vi "DuelistDirectIndirect.vi"(8 "error in (no error)":errorcluster, 10 "Game in":refnum<class "Game.lvclass">, 11 "NormalDefensiveWithDuelistPlay in":refnum<class "NormalDefensiveWithDuelistPlay.lvclass">) -> (0 "error out":errorcluster, 2 "duelist ?":bool, 3 "NormalDefensiveWithDuelistPlay out":refnum<class "NormalDefensiveWithDuelistPlay.lvclass">)   [LabVIEW 2018, in "NormalDefensiveWithDuelistPlay.lvclass"]
uses:
  NormalDefensiveWithDuelistPlay.lvclass
  Game_class/Game.lvclass
  Referee_class/command_interpreted.ctl
  Game_class/Game.lvclass/Game.ctl
  Referee_class/Referee.lvclass/Referee.ctl
  Events_class/Events.lvclass/Events.ctl
  Game_class/Read Referee.vi
  Game_class/Read EventsRef.vi
  Events_class/Read touch.vi
  Referee_class/Read command_interpreted.vi
  Referee_class/Referee.lvclass
  Events_class/Events.lvclass
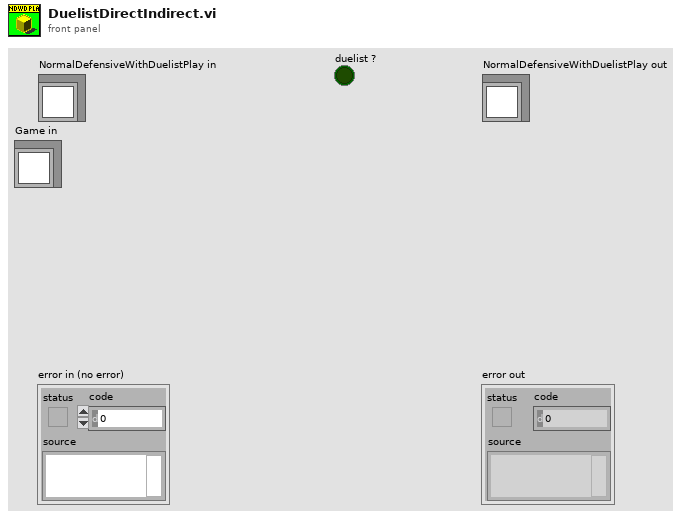
[diagram p1: front panel]
types:
  T1 = typedef "command_interpreted.ctl" = enum16{"Goal Ally", "Goal Enemy", "Ball Placement Enemy", "Ball Placement Ally", "Normal Half Time", "Extra Time  Break", "Extra Half Time", "None", "Post Game", "PKA Normal Start", "Prepare Kickoff Ally", "PKE Normal Start", "Prepare Kickoff Enemy", "Force Start", "Halt", "Timeout", "Prepare Penalty Ally", "Prepare Penalty Enemy", "PPA NormalStart", "PPE Normal Start", "Indirect Free Ally", "Direct Free Enemy", "Direct Free Ally", "Indirect Free Enemy", "Stop"}
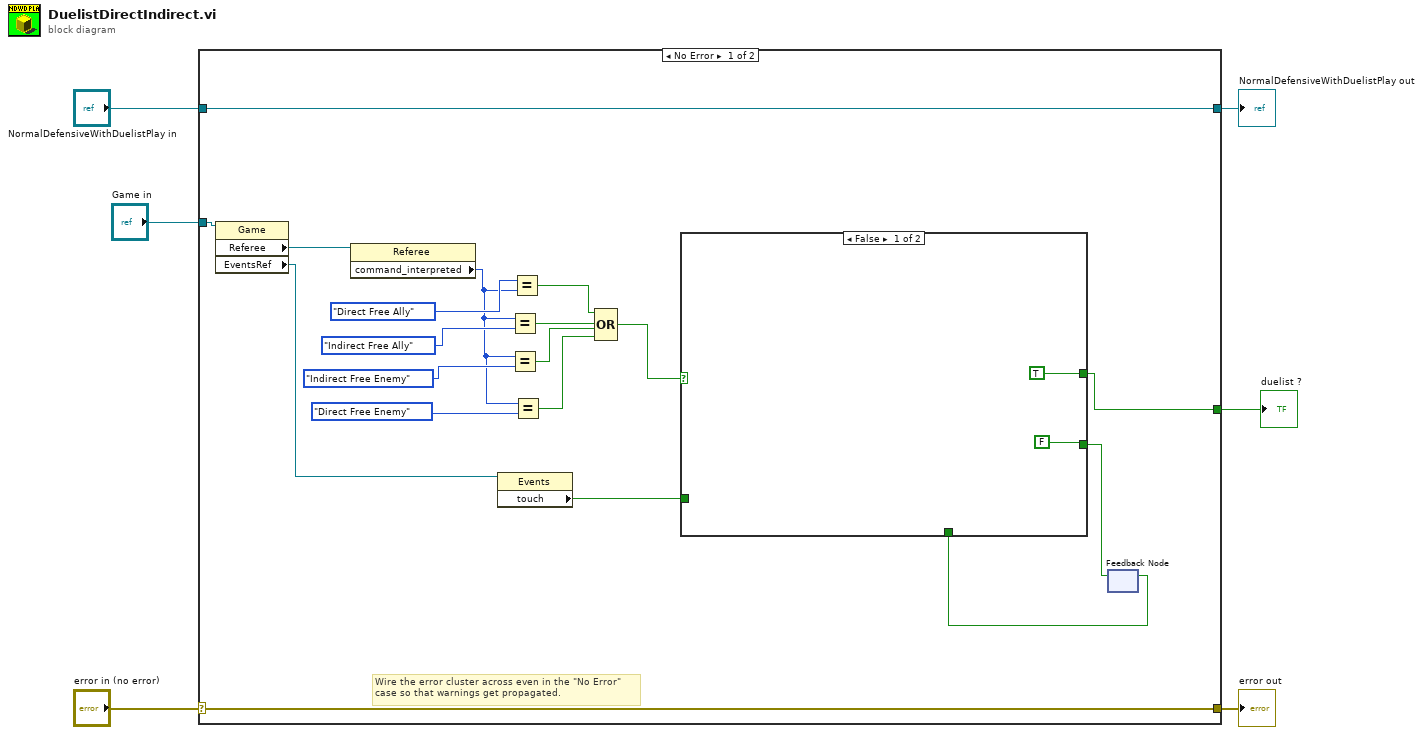
[diagram p0: block diagram]
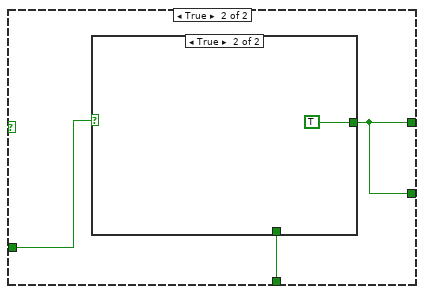
[diagram p2: hidden frame]
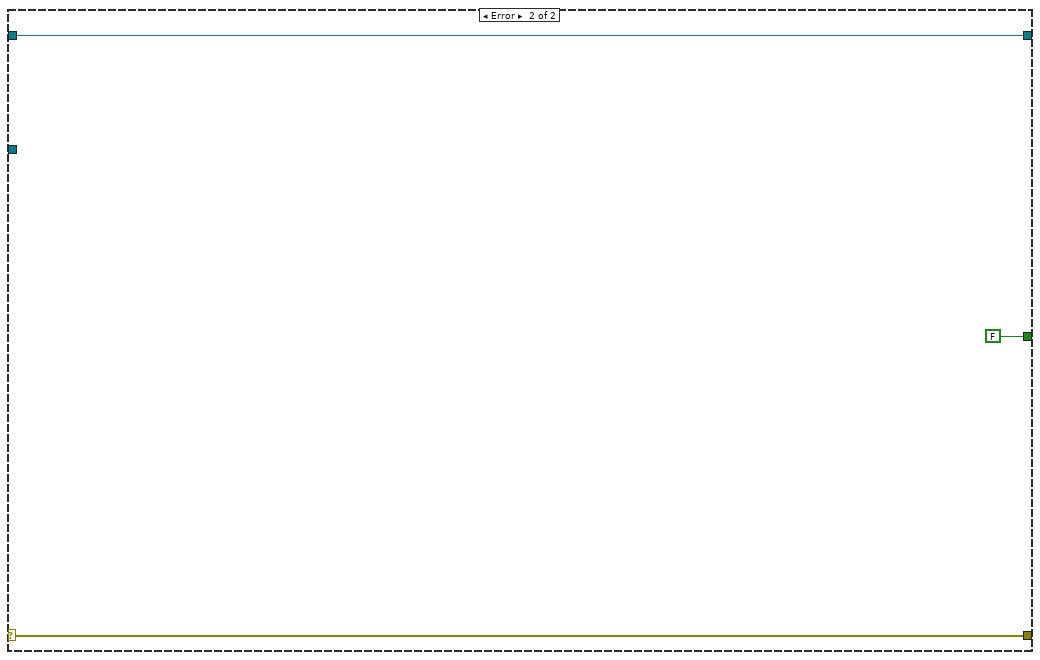
[diagram p4: hidden frame]
diagram:
  n1 = case shown="No Error" "error in (no error)" {
    selector: "error in (no error)" -> [w24 w35]
    tunnel: [w24 w35] -> w5
    tunnel: [w25 w34] -> w3
    tunnel: "NormalDefensiveWithDuelistPlay in" -> [w25 w34]
    tunnel: "Game in" -> [w23 _]
    tunnel: [w8 FALSE] -> w1
    frame No Error {
      # "Wire the error cluster across even in the \"No Error\"\ncase so that warnings get propagated."
      n2 = property class="Game"(reference=w23) -> ("Referee"=w22:refnum<class "Referee.lvclass">, "EventsRef"=w12:refnum<class "Events.lvclass">)  [unwired: 1 in, 2 out]
      n3 = property class="Referee"(reference=w22) -> ("command_interpreted"=w17:T1)  [unwired: 1 in, 2 out]
      n4 = property class="Events"(reference=w12) -> ("touch"=w10:bool)  [unwired: 1 in, 2 out]
      n5 = Equal?(x=w17, y=command_interpreted."Indirect Free Ally") -> (x = y?=w15:bool)
      n6 = Equal?(x=w17, y=command_interpreted."Indirect Free Enemy") -> (x = y?=w14:bool)
      n7 = Equal?(x=command_interpreted."Direct Free Ally" ("y"), y=w17) -> (x = y?=w16:bool)
      n8 = Equal?(x=w17, y=command_interpreted."Direct Free Enemy") -> (x = y?=w13:bool)
      n9 = Compound Arithmetic op=OR(w16, w15, w14, w13) -> (w11:bool)
      n10 = feedback #1() -> (w9:bool)  [unwired: 1 in]
      n11 = case shown="False" w11 {
        tunnel: w10 -> [_ w30]
        tunnel: [TRUE w28] -> w8
        tunnel: w9 -> [_ w29]
        tunnel: [FALSE w28] -> w7
        frame False {
        }
        frame True {
          n12 = case shown="True" w30 {
            tunnel: [w31 TRUE] -> w28
            tunnel: w29 -> [w31 _]
            frame False {
            }
            frame True {
            }
          }
        }
      }
      n13 = feedback-in #1(w7) -> ()
    }
    frame Error {
    }
  }
  "error out" <- w5
  "NormalDefensiveWithDuelistPlay out" <- w3
  "duelist ?" <- w1
